vi "TSM SSC Digital N Pins To M Sessions.vi"(0 "TSM context":T3, 1 "Turn Pin Groups to Pins?":bool=TRUE caption="Turn Pin Groups to Pins? (T)", 5 "Pins":tag[](array[tag]), 7 "Site Numbers":i32[](array[numeric]), 11 "error in":errorcluster) -> (4 "Digital TSM Out":T1, 15 "error out":errorcluster)   [LabVIEW 2019]
doc: "Populates the TSM SSC Digital cluster for the specified pin(s) and pin group(s). \n\nThe \"Turn Pin Groups to Pins?\" should be set to TRUE when using pin groups, since it's important for the TSM SSC functions to have a full list of DUT pins when mapping instrument indexed results into per-site per-pin results.\n\nThe \"Turn Pin Groups to Pins?\" input can be set to FALSE <b>if the Pins input doesn't contain any pin groups</b>. This setting is preferred when optimizing test time."
uses:
  <vilib>/NI_TestStand_SemiconductorModule/NI_TestStand_Semiconductor_Module.lvlibp/PinMap/General/SemiconductorModuleContext.ctl
  TSM SSC Digital.ctl
  <vilib>/NI_TestStand_SemiconductorModule/NI_TestStand_Semiconductor_Module.lvlibp/PinMap/Digital Pattern/PinQueryContext/DigitalPatternPinQueryContext.lvclass
  SSC Digital/SSC Digital.ctl
  <vilib>/NI_TestStand_SemiconductorModule/NI_TestStand_Semiconductor_Module.lvlibp/PinMap/Advanced/GetPinsInPinGroups.vi
  <vilib>/NI_TestStand_SemiconductorModule/NI_TestStand_Semiconductor_Module.lvlibp/PinMap/Digital Pattern/PinsToNIDigitalPatternSessions.vi
  <vilib>/NI_TestStand_SemiconductorModule/NI_TestStand_Semiconductor_Module.lvlibp
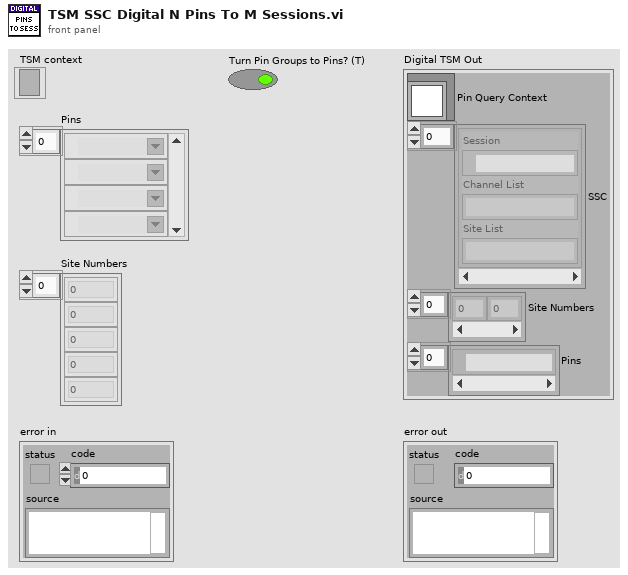
[diagram p1: front panel]
types:
  T1 = typedef "TSM SSC Digital.ctl" = cluster{"Pin Query Context":refnum<class "DigitalPatternPinQueryContext.lvclass">, "SSC":T2[], "Site Numbers":i32[], "Pins":tag[]}
  T2 = typedef "SSC Digital.ctl" = cluster{"Session":refnum<k15>, "Channel List":string, "Site List":string}
  T3 = typedef "NI_TestStand_Semiconductor_Module.lvlibp/SemiconductorModuleContext.ctl" = refnum<k7>
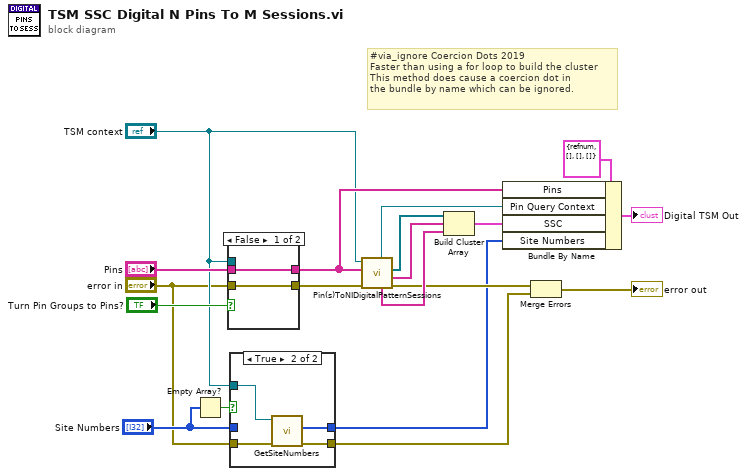
[diagram p0: block diagram]
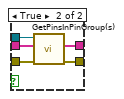
[diagram p3: hidden frame]
diagram:
  # "#via_ignore Coercion Dots 2019\nFaster than using a for loop to build the cluster\nThis method does cause a coercion dot in\nthe bundle by name which can be ignored."
  n1 = Empty Array?(array="Site Numbers") -> (empty?=w5:bool)
  n2 = case shown="False" "Turn Pin Groups to Pins?" {
    tunnel: "error in" -> [w20 w26]
    tunnel: [w20 w25] -> w12
    tunnel: "TSM context" -> [_ w24]
    tunnel: "Pins" -> [w21 w23]
    tunnel: [w21 w22] -> w10
    frame False {
    }
    frame True {
      n3 = call-poly <vilib>:"GetPinsInPinGroup(s).vi"("error in (no error)"=w26, "Pin Groups"=w23, "Semiconductor Module Context"=w24) -> ("error out"=w25:errorcluster, "Pins"=w22:tag[])  [unwired: 6 in, 1 out]
    }
  }
  n4 = case shown="True" w5 {
    tunnel: "error in" -> [w27 w32]
    tunnel: [w27 w31] -> w1
    tunnel: "TSM context" -> [_ w30]
    tunnel: [w28 w29] -> w7
    tunnel: "Site Numbers" -> [w28 _]
    frame False {
    }
    frame True {
      n5 = call <vilib>:"GetSiteNumbers.vi"("error in (no error)"=w32, "Semiconductor Module Context"=w30) -> ("error out"=w31:errorcluster, "Site Numbers"=w29:i32[])  [unwired: 6 in, 2 out]
    }
  }
  n6 = call-poly <vilib>:"Pin(s)ToNIDigitalPatternSessions.vi"("error in (no error)"=w12, "Pins"=w10, "Semiconductor Module Context"="TSM context") -> ("error out"=w9:errorcluster, "Channel Lists"=w15:string[], "Instrument Sessions"=w16:refnum<k15>[], "Site Lists"=w14:string[], "Pin Query Context"=w18:refnum<class "DigitalPatternPinQueryContext.lvclass">)  [unwired: 3 in, 1 out]
  n7 = Build Cluster Array(w16, w15, w14) -> (w13:cluster{refnum<k15>, string, string}[])
  n8 = Bundle By Name(cluster=T1 {"Pin Query Context"=refnum, "SSC"=[], "Site Numbers"=[], "Pins"=[]} ("DAQmx - Multiple Sessions Info"), "Pins"=w10, "Pin Query Context"=w18, "SSC"=w13, "Site Numbers"=w7) -> (→"Digital TSM Out":T1)
  n9 = Merge Errors(w9, w1) -> (→"error out":errorcluster)
